vi "Main RT V2.vi"() -> ()   [LabVIEW 2010]
uses:
  RT Code Modules/RT Tritech Sonar Module/RT Tritech Sonar Module Controls.ctl
  RT Code Modules/RT Tritech Sonar Module/SeaNet Protocol Utilities/SeaNet Head Control.ctl
  RT Code Modules/RT Tritech Sonar Module/SeaNet Protocol Utilities/SeaNet Motor Data.ctl
  RT Code Modules/RT Tritech Sonar Module/SeaNet Protocol Utilities/SeaNet Range Data.ctl
  RT Code Modules/RT Tritech Sonar Module/RT Tritech Sonar Module Indicators.ctl
  FPGA Code/Modules/Tritech Sonar Module/Internal Type Defs/FPGA Tritech Read Write State.ctl
  FPGA Code/Modules/Tritech Sonar Module/Internal Type Defs/FPGA Tritech Error Cluster.ctl
  FPGA Code/Modules/Tritech Sonar Module/Internal Type Defs/FPGA Tritech Error Enumeration.ctl
  FPGA Code/Modules/Tritech Sonar Module/Self Test FSM/FPGA Tritech Self Test FSM State.ctl
  FPGA Code/Modules/Tritech Sonar Module/Self Test FSM/FPGA Tritech Self Test FSM Memory.ctl
  FPGA Code/Modules/Tritech Sonar Module/Internal Type Defs/FPGA Tritech Self TD.ctl
  FPGA Code/Modules/Tritech Sonar Module/Superficial Parser FSM/FPGA Tritech Superficial Parser FSM State.ctl
  FPGA Code/Modules/Tritech Sonar Module/Superficial Parser FSM/FPGA Tritech Superficial Parser FSM Mem.ctl
  FPGA Code/Modules/Tritech Sonar Module/Tritech Utilities/Tritech mtEnum.ctl
  FPGA Code/Modules/Utilities/Data Latch.ctl
  RT Code Modules/RT Tritech Sonar Module/SeaNet Protocol Utilities/SeaNet Head Inf.ctl
  RT Code Modules/RT Tritech Sonar Module/SeaNet Protocol Utilities/SeaNet mtHeadData Information.ctl
  RT Code Modules/RT Tritech Sonar Module/SeaNet Protocol Utilities/SeaNet Head Status.ctl
  RT Code Modules/RT Tritech Sonar Module/SeaNet Protocol Utilities/SeaNet Sweep Code.ctl
  RT Code Modules/RT Tritech Sonar Module/Think/RT Think Waveform Graph.ctl
  RT Code Modules/RT Finset Module/RT Finset Module Controls.ctl
  RT Code Modules/RT Finset Module/RT Finset Module Indicators.ctl
  <vilib>/rvi/interface/nirviReadWriteControl/nirviReadWriteControl.xnode
  FPGA Interface.ctl
  FPGA Bitfiles/FishArchitecture_FPGATarget_MainFPGAV2_487E23F7.lvbitx
  FPGA Code/Main FPGA V2.vi
  <vilib>/rvi/interface/common/niFpgaNodeNameForErrorReporting.ctl
  <vilib>/rvi/errors/niLvFpgaWhatHappensToTopLevelVI.ctl
  <vilib>/rvi/interface/nirviCloseFPGA/nirviCloseFPGA.xnode
  <vilib>/Utility/error.llb/Error Cluster From Error Code.vi
  <vilib>/rvi/errors/niLvFpgaAdjustHostInterfaceError.vi
  <vilib>/FPGAPlugInAG/cRIO-9073/niLvFpga_Close_cRIO-9073.vi
  NiFpgaLv.dll
panel:
  in  "Restart":bool
  out "HB":bool caption="Heart Beat"
  in  "stop":bool
  in  "Main GUI Tabs":T1(tab)
  out "Tritech Indicators":T2={"LRW FSM State"=enum."Write", "FPGA Read Error"={"Error"=FALSE, "Error Type"=enum."No Error"}, "Self Test FSM State"=enum."Wait to Finish Reading mtAlive", "Self Test FSM Memory"={"Previous State"=enum."Wait to Finish Reading mtAlive", "Timeout counter"=0, "Counter"=0, "Special Purpose Failure Counter"=0, "Previous Failed State"=enum."Wait to Finish Reading mtAlive", "Message Seems Legit"=TRUE, "Current State"={"mtAlive Received"=FALSE, "mtVersionData Received"=FALSE}, "1 Min Timer (ms)"=0, "First Failure"=enum."Wait to Finish Reading mtAlive", "Which States Have Failed?"=[FALSE, FALSE, FALSE, FALSE, FALSE, FALSE, FALSE, FALSE, FALSE, FALSE, FALSE]}, "Superficial Parser FSM"={"State"=enum."Wait for Start", "Memory"={"Index"=0, "Hex Message Size"=0, "AXCIIHex Message Size"=0, "Message Enum"=enum."mtSendPerformanceData", "Master Index"=0}}, "Messages Received"=[], "Messages Sent"=[], "FPGA"=[], "RT"=[], "Head Inf"={"In Centre"=FALSE, "Centered"=FALSE, "Motoring"=FALSE, "Motor On"=FALSE, "Dir"=FALSE, "In Scan"=FALSE, "No Params"=FALSE, "SendCfg"=FALSE}, "Head Position"=0, "Head Time"=0, "mtHeadData"={"R-Limit"=0, "L-Limit"=0, "Bearing"=0, "Dbytes"=0, "Steps"=0, "Head Status"={"HdPwrLoss"=FALSE, "MotErr"=FALSE, "PrfSyncErr"=FALSE, "PrfPingErr"=FALSE, "8BitMode"=FALSE, "Ignoreme"=FALSE, "Ignoreme2"=FALSE, "MesAppnd"=FALSE}, "Sweep Code"={"Scanning Normal"=FALSE, "Scan_AtLeftLimit"=FALSE, "Scan_AtRightLimit"=FALSE, "Ignore1"=FALSE, "Ignore2"=FALSE, "Scan_AtCentre"=FALSE, "Ignore3"=FALSE, "Ignore4"=FALSE}, "Range Scale"=0, "AD Span"=0, "Gain"=0, "Head Control"={"Use 8 bit ADC (4 bit)"=FALSE, "Continuous Rotoation (Sector Scan)"=FALSE, "Scan Right (Scan Left)"=FALSE, "Upside down (Rightside up)"=FALSE, "Motor off (Motor On)"=FALSE, "Transmit Off (On)"=FALSE, "Apply Heading Offset (Ignore)"=FALSE, "Ping Pong (Don't)"=FALSE}}, "Waveform Graph"=[]} {"mtHeadData"."Bearing" format="%.0x"; "mtHeadData"."L-Limit" format="%.0x"; "mtHeadData"."R-Limit" format="%.0x"; "Self Test FSM Memory"."1 Min Timer (ms)" format="%x"}
  in  "Tritech Commands":T19={"Send Error Ack"=FALSE, "Manual Override"=FALSE, "Sweep Select"=enum."360 Sweep", "Turn Curvature"=0.0, "Manual Message"="", "Manual"=FALSE, "Easy Message"="", "Easy"=FALSE, "Cheating Message"=enum."mtReboot", "Cheating!"=FALSE, "Head Control"={"Use 8 bit ADC (4 bit)"=FALSE, "Continuous Rotoation (Sector Scan)"=FALSE, "Scan Right (Scan Left)"=FALSE, "Upside down (Rightside up)"=FALSE, "Motor off (Motor On)"=FALSE, "Transmit Off (On)"=FALSE, "Apply Heading Offset (Ignore)"=FALSE, "Ping Pong (Don't)"=FALSE}, "Motor"={"Step Size"=32, "LeftLim"=1, "RightLim"=6399, "Motor Time"=25}, "Range"={"ADSpan"=77, "ADLow"=40, "ADInterval"=104, "Nbins"=200, "IGain"=84, "RangeScale"=60}} {"Motor"."Step Size" format="%.0x"; "Motor"."Motor Time" format="%.0x"; "Motor"."RightLim" format="%.0x"; "Motor"."LeftLim" format="%.0x"}
  out "Finset Indicators":T22
  in  "Finset Commands":T23
  # "We have stuff to do in terms of the plotting.\nand by we I mean me.\n\nI broke the plotter, bythe way.\nThere is good data in there, but I'm remaking\nthe array every time."
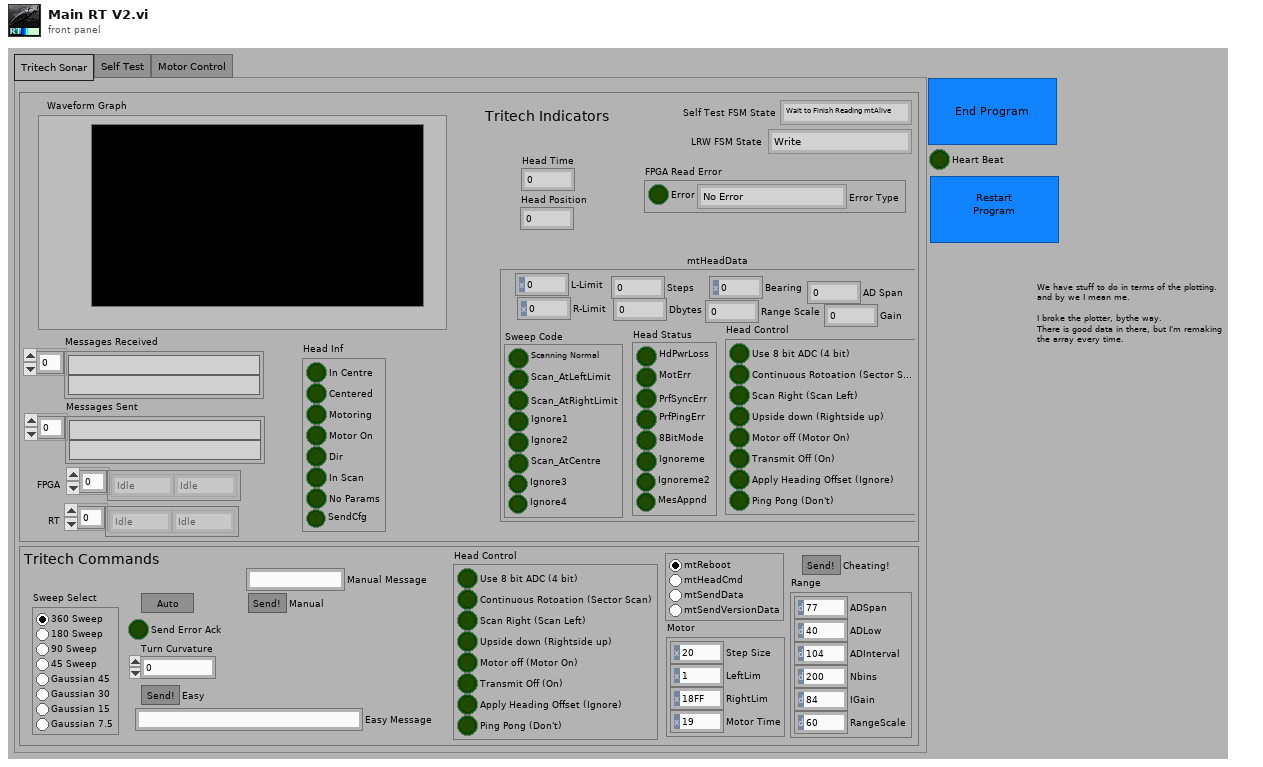
[diagram p1: front panel]
types:
  T1 = enum32{"Tritech Sonar", "Self Test", "Motor Control"}
  T2 = typedef "RT Tritech Sonar Module Indicators.ctl" = cluster{"LRW FSM State":T3, "FPGA Read Error":T4, "Self Test FSM State":T6, "Self Test FSM Memory":T7, "Superficial Parser FSM":cluster{"State":T9, "Memory":T10}, "Messages Received":string[], "Messages Sent":string[], "FPGA":T12[], "RT":T12[], "Head Inf":T13, "Head Position":u16, "Head Time":u32, "mtHeadData":T14, "Waveform Graph":T18}
  T3 = typedef "FPGA Tritech Read Write State.ctl" = enum16{"Write", "Read"}
  T4 = typedef "FPGA Tritech Error Cluster.ctl" = cluster{"Error":bool, "Error Type":T5}
  T5 = typedef "FPGA Tritech Error Enumeration.ctl" = enum8{"No Error", "Unexpected Line Feed", "Message Over Bounds", "Sizes Disagree: First Hex", "Sizes Disagree: Second Hex", "Unexpected Sender", "Unexpected Receiver", "Send Recive Inconsistant", "Unknown Message Type", "ASCIIHex: Bad Charactor", "Double '@' Header", "u8 FIFO to RT Timeout", "Master Timeout"}
  T6 = typedef "FPGA Tritech Self Test FSM State.ctl" = enum8{"Wait to Finish Reading mtAlive", "Compare to mtAlive", "Write mtSendVersion to Buffer", "Switch to Write Mode", "Wait for Write to Finish", "Wait for Reply", "Compare Reply to mtVersionData", "Handle Success", "Handle Failure"}
  T7 = typedef "FPGA Tritech Self Test FSM Memory.ctl" = cluster{"Previous State":T6, "Timeout counter":u16, "Counter":u16, "Special Purpose Failure Counter":u16, "Previous Failed State":T6, "Message Seems Legit":bool, "Current State":T8, "1 Min Timer (ms)":u16, "First Failure":T6, "Which States Have Failed?":bool[]}
  T8 = typedef "FPGA Tritech Self TD.ctl" = cluster{"mtAlive Received":bool, "mtVersionData Received":bool}
  T9 = typedef "FPGA Tritech Superficial Parser FSM State.ctl" = enum16{"Wait for Start", "Read ASCIIhex length", "Read Hex Length", "Read Sender", "Read Recipient", "Read Byte Count", "Read Message Type", "Wait for Message to End", "Confirm Finish"}
  T10 = typedef "FPGA Tritech Superficial Parser FSM Mem.ctl" = cluster{"Index":u16, "Hex Message Size":u16, "AXCIIHex Message Size":u16, "Message Enum":T11, "Master Index":u16}
  T11 = typedef "Tritech mtEnum.ctl" = enum8{"mtNull", "mtVersionData", "mtHeadData", "mtSpectData", "mtAlive", "mtPrgAck", "mtBBUserData", "mtTestData", "mtAuxData", "mtAdcData", "mtAdcReq", "Void 11", "Void 12", "mtLanStatus", "mtSetTime", "mtTimeout", "mtReboot", "mtPerformanceData", "Void 18", "mtHeadCommand", "mtEraseSector", "mtProgBlock", "mtCopyBootBlk", "mtSendVersion", "mtSendBBuser", "mtSendData", "mtSendPerformanceData"}
  T12 = typedef "Data Latch.ctl" = enum8{"Idle", "Sending", "Sent", "Receiving", "Received"}
  T13 = typedef "SeaNet Head Inf.ctl" = cluster{"In Centre":bool, "Centered":bool, "Motoring":bool, "Motor On":bool, "Dir":bool, "In Scan":bool, "No Params":bool, "SendCfg":bool}
  T14 = typedef "SeaNet mtHeadData Information.ctl" = cluster{"R-Limit":u16, "L-Limit":u16, "Bearing":u16, "Dbytes":u16, "Steps":u8, "Head Status":T15, "Sweep Code":T16, "Range Scale":u16, "AD Span":u8, "Gain":u8, "Head Control":T17}
  T15 = typedef "SeaNet Head Status.ctl" = cluster{"HdPwrLoss":bool, "MotErr":bool, "PrfSyncErr":bool, "PrfPingErr":bool, "8BitMode":bool, "Ignoreme":bool, "Ignoreme2":bool, "MesAppnd":bool}
  T16 = typedef "SeaNet Sweep Code.ctl" = cluster{"Scanning Normal":bool, "Scan_AtLeftLimit":bool, "Scan_AtRightLimit":bool, "Ignore1":bool, "Ignore2":bool, "Scan_AtCentre":bool, "Ignore3":bool, "Ignore4":bool}
  T17 = typedef "SeaNet Head Control.ctl" = cluster{"Use 8 bit ADC (4 bit)":bool, "Continuous Rotoation (Sector Scan)":bool, "Scan Right (Scan Left)":bool, "Upside down (Rightside up)":bool, "Motor off (Motor On)":bool, "Transmit Off (On)":bool, "Apply Heading Offset (Ignore)":bool, "Ping Pong (Don't)":bool}
  T18 = typedef "RT Think Waveform Graph.ctl" = dbl[][]
  T19 = typedef "RT Tritech Sonar Module Controls.ctl" = cluster{"Send Error Ack":bool, "Manual Override":bool, "Sweep Select":enum32{"360 Sweep", "180 Sweep", "90 Sweep", "45 Sweep", "Gaussian 45", "Gaussian 30", "Gaussian 15", "Gaussian 7.5"}, "Turn Curvature":dbl, "Manual Message":string, "Manual":bool, "Easy Message":string, "Easy":bool, "Cheating Message":enum32{"mtReboot", "mtHeadCmd", "mtSendData", "mtSendVersionData"}, "Cheating!":bool, "Head Control":T17, "Motor":T20, "Range":T21}
  T20 = typedef "SeaNet Motor Data.ctl" = cluster{"Step Size":u8, "LeftLim":u16, "RightLim":u16, "Motor Time":u8}
  T21 = typedef "SeaNet Range Data.ctl" = cluster{"ADSpan":u8, "ADLow":u8, "ADInterval":u16, "Nbins":u16, "IGain":u8, "RangeScale":u16}
  T22 = typedef "RT Finset Module Indicators.ctl" = cluster{"Messages Received":string[], "Messages Sent":string[], "FPGA":T12[], "RT":T12[]}
  T23 = typedef "RT Finset Module Controls.ctl" = cluster{"Message":string, "Send":bool, "Append LF/CR?":bool, "Initialize":bool, "Stop":bool, "Command type":enum16{"Manual", "Absolute position", "Forward", "Reverse", "Query", "Set position", "Set encoder ratio", "Set run current", "Set hold current"}}
  T24 = typedef "niFpgaNodeNameForErrorReporting.ctl" = enum16{"Open FPGA VI Reference", "Read/Write Control", "Invoke Method: Abort", "Invoke Method: Acknowledge IRQ", "Invoke Method: Download", "Invoke Method: FIFO.Configure", "Invoke Method: FIFO.Read", "Invoke Method: FIFO.Start", "Invoke Method: FIFO.Stop", "Invoke Method: FIFO.Write", "Invoke Method: Reset", "Invoke Method: Run", "Invoke Method: Wait on IRQ", "Close FPGA VI Reference"}
  T25 = typedef "niLvFpgaWhatHappensToTopLevelVI.ctl" = enum16{"top level VI scripted behind XNode", "top level VI inlined behind XNode"}
  T26 = typedef "FPGA Interface Queue.ctl" = refnum<queue>
  T27 = typedef "FPGA Interface.ctl" = refnum<k20>
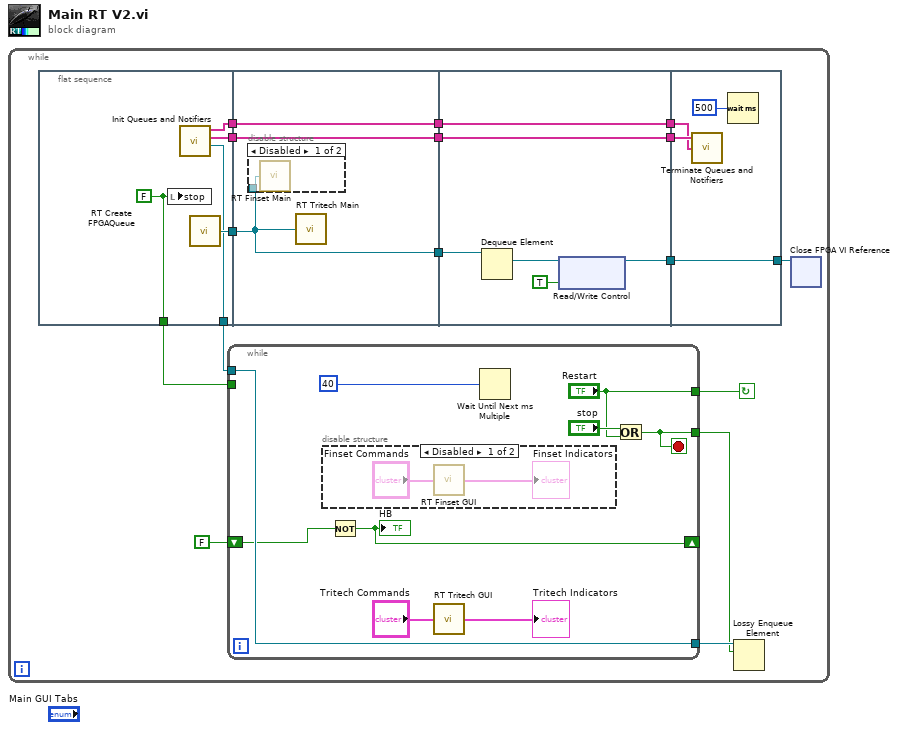
[diagram p0: block diagram]
diagram:
  n1 = while {
    stop <- w11 continue-if-true
    n2 = flat-sequence {
      tunnel: [w27] -> w15
      tunnel: [w26] -> w16
      tunnel: [w25] -> w12
      tunnel: [w24] -> w7
      tunnel: [w23] -> w4
      tunnel: w16 -> [w30]
      tunnel: [w30] -> w10
      tunnel: w7 -> [w29]
      tunnel: [w29] -> w6
      tunnel: w4 -> [w28]
      tunnel: [w28] -> w3
      tunnel: w10 -> [w37]
      tunnel: [w34] -> w9
      tunnel: w6 -> [w33]
      tunnel: [w33] -> w5
      tunnel: w3 -> [w32]
      tunnel: [w32] -> w2
      tunnel: w9 -> [w78]
      tunnel: [w78] -> w8
      tunnel: w5 -> [w77]
      tunnel: w2 -> [w76]
      frame #0 {
        w27 = FALSE ("stop")
        n3 = local write "stop"(w27) -> ()
        n4 = call "Init Queues and Notifiers.vi"() -> ("Shutdown Queue"=w25:refnum<queue>, "List of All Notifier Names"=w24:string[], "List of All Queue Names"=w23:string[])  [unwired: 7 in, 2 out]
        n5 = call "RT Create FPGAQueue.vi"() -> ("queue out"=w26:T26)
      }
      frame #1 {
        n6 = disable-structure shown="Disabled" {
          disable-tunnel: w30 -> [w31 _]
          frame Disabled {
            n7 = call "RT Finset Main.vi"("FPGA Interface in"=w31) -> ()  [unwired: 1 in]
          }
          frame Enabled {
          }
        }
        n8 = call "RT Tritech Main.vi"("FPGA Reference"=w30) -> ()
      }
      frame #2 {
        n9 = Dequeue Element(queue=w37) -> (element=w35:T27)  [unwired: 2 in, 3 out]
        n10 = xnode "Read/Write Control"("FPGA VI Reference In"=w35, "Shutdown"=TRUE) -> ("FPGA VI Reference Out"=w34:T27)  [unwired: 1 in, 1 out]
      }
      frame #3 {
        n11 = call "Terminate Queues and Notifiers.vi"("List of All Queue Names"=w76, "List of All Notifier Names"=w77) -> ()  [unwired: 3 in, 1 out]
        n12 = Wait (ms)(milliseconds to wait=u32 500) -> ()  [unwired: 1 out]
      }
    }
    n13 = while {
      tunnel: w15 -> [_]
      tunnel: [w87] -> w14
      tunnel: w12 -> [w87]
      tunnel: [w85] -> w13
      tunnel: ["Restart"] -> w11
      shift-right: [w83] -> _
      shift-left: FALSE -> [w82]
      stop <- w85 stop-if-true
      n14 = disable-structure shown="Disabled" {
        frame Disabled {
          n15 = call "RT Finset GUI.vi"("Finset Commands"="Finset Commands") -> ("Finset Indicators"=→"Finset Indicators":T22)
        }
        frame Enabled {
        }
      }
      n16 = Not(x=w82) -> (.not. x?=w83:bool)
      "HB" <- w83
      n17 = call "RT Tritech GUI.vi"("Tritech Commands"="Tritech Commands") -> ("Tritech Indicators"=→"Tritech Indicators":T2)
      n18 = Wait Until Next ms Multiple(millisecond multiple=u32 40) -> ()  [unwired: 1 out]
      n19 = Or(x="stop", y="Restart") -> (x .or. y?=w85:bool)
    }
    n20 = Lossy Enqueue Element(queue=w14, element=w13) -> ()  [unwired: 1 in, 4 out]
    n21 = xnode "Close FPGA VI Reference"("FPGA VI Reference In"=w8) -> ()  [unwired: 1 in, 1 out]
  }
